vi "Log to Excel.vi"(8 "error in":errorcluster, 11 "tdms file in":refnum<k34>) -> (0 "error out":errorcluster, 2 "appended array":dbl[][][](array[numeric]), 3 "tdms file out":refnum<k34>)   [LabVIEW 2015, in "Logger.lvlib"]
uses:
  Logger.lvlib
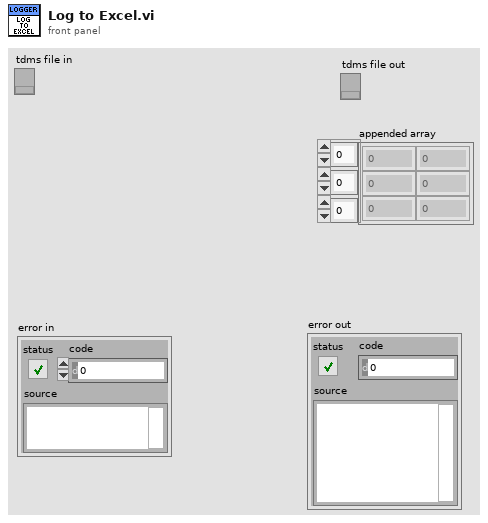
[diagram p1: front panel]
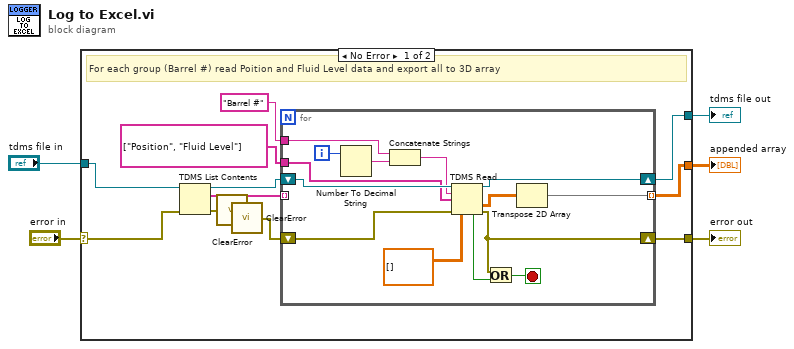
[diagram p0: block diagram]
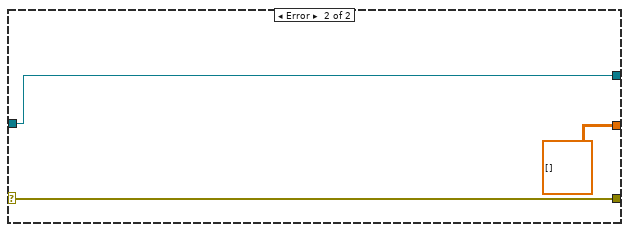
[diagram p2: hidden frame]
diagram:
  n1 = case shown="No Error" "error in" {
    selector: "error in" -> [w11 w34]
    tunnel: [w16 dbl[][][] []] -> w5
    tunnel: [w15 w34] -> w4
    tunnel: [w13 w33] -> w3
    tunnel: "tdms file in" -> [w8 w33]
    frame No Error {
      # "For each group (Barrel #) read Poition and Fluid Level data and export all to 3D array"
      n2 = TDMS List Contents(4:w11, 7:w8) -> (0:w6:errorcluster, 2:w12:string[], 3:w9:refnum<k34>)  [unwired: 1 in, 1 out]
      n3 = call <vilib>:"ClearError.vi"("error in (no error)"=w6) -> ("error out"=w7:errorcluster)
      n4 = call <vilib>:"ClearError.vi"("error in (no error)"=w7) -> ("error out"=w10:errorcluster)
      n5 = for {
        tunnel: string[] ["Position", "Fluid Level"] -> [w23]
        tunnel: "Barrel #" -> [w28]
        tunnel: [w21] -> w16 mode=indexing
        shift-right: [w20] -> w15
        shift-left: w10 -> [w30]
        tunnel: w12 -> [_] mode=indexing
        shift-right: [w25] -> w13
        shift-left: w9 -> [w31]
        i -> [w26]
        stop <- w18 stop-if-true
        n6 = Number To Decimal String(number=w26) -> (decimal integer string=w27:string)  [unwired: 1 in]
        n7 = Concatenate Strings(w28, w27) -> (w24:string)
        n8 = TDMS Read(0:w31, 5:w24, 7:w23, 11:w30, 12:dbl[][] [] ("appended array")) -> (4:w25:refnum<k34>, 10:w22:dbl[][], 14:w19:bool, 15:w20:errorcluster)  [unwired: 3 in, 2 out]
        n9 = Or(x=w20, y=w19) -> (x .or. y?=w18:bool)
        n10 = Transpose 2D Array(2D array=w22) -> (transposed array=w21:dbl[][])
      }
    }
    frame Error {
    }
  }
  "error out" <- w4
  "appended array" <- w5
  "tdms file out" <- w3
